vi "Read database.vi"(0 "table":string="CODMn", 1 "显示项":string[](array[string]), 5 "量程下拉列表":enum16{"低量程", "高量程"}(ring), 11 "error in (no error)":errorcluster caption="错误输入（无错误）") -> (4 "表格":string[][](table), 8 "foretime":string, 10 "lasttime":string, 15 "error out":errorcluster caption="错误输出")   [LabVIEW 2016, in "斯坦道CODcr.lvlib"]
uses:
  <vilib>/addons/database/Connection.llb/DB Tools Open Connec (String).vi
  <vilib>/addons/database/_DB Variant To Data/Database Variant To Data.xnode
  <vilib>/addons/database/NI_Database_API.lvlib
  database/SQLite/SQLite Lib.lvlib
  database/Access/Access Lib.lvlib
panel:
  out "电子表格字符串":string
  out "SQL":string="where 时间 between #2020/03/27 14:26:18 # and #2020/04/26 14:26:18# order by 时间 desc"
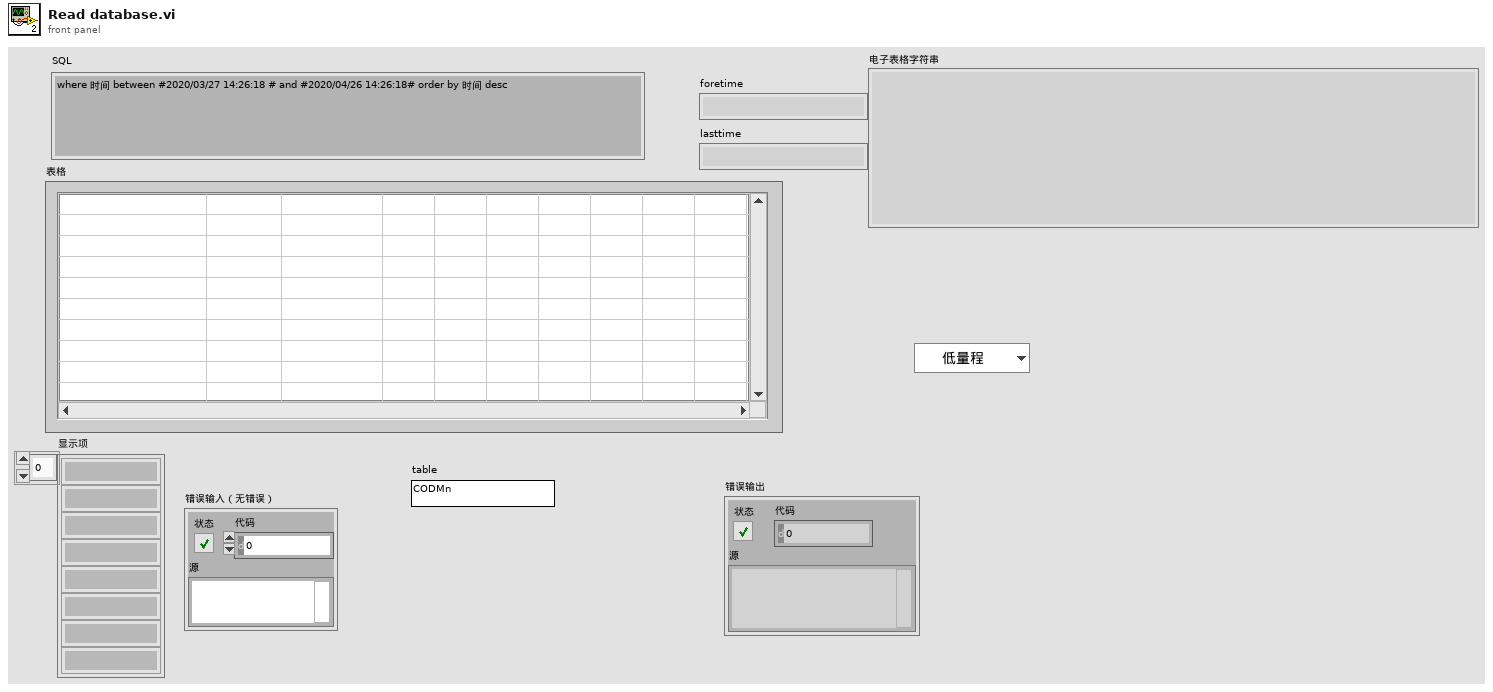
[diagram p1: front panel]
types:
  T1 = typedef "数据库类型.ctl" = enum16{"Access", "SQLite"}
  T2 = typedef "NI_Database_API.lvlib/Conn ObjectReference.ctl" = refnum<k1>
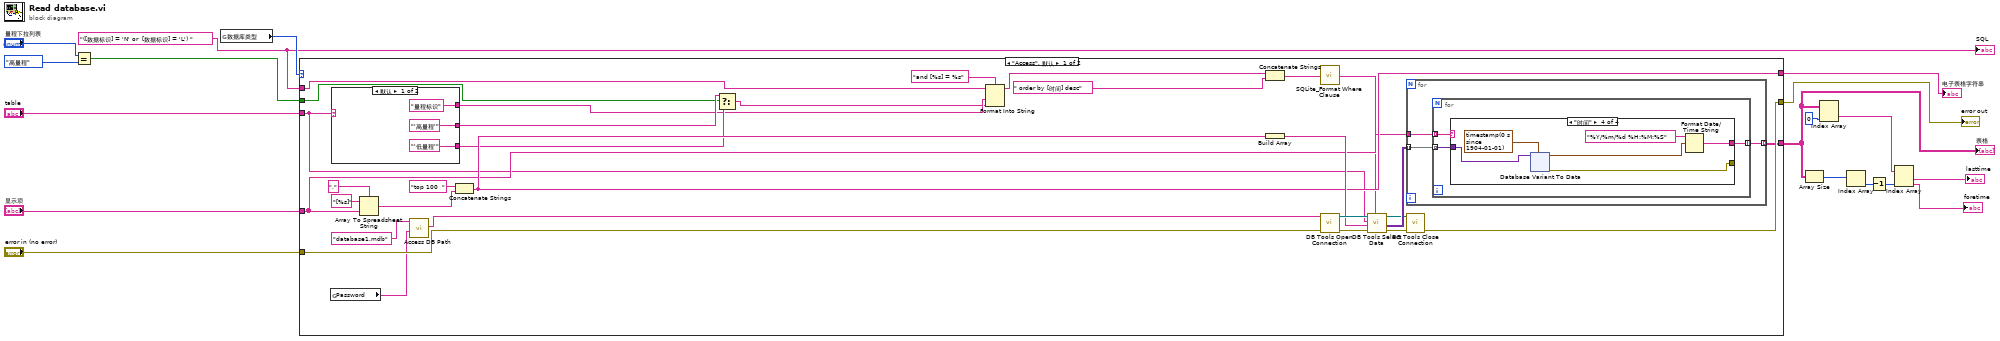
[diagram p0: block diagram]
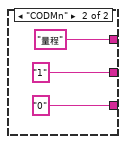
[diagram p2: hidden frame]
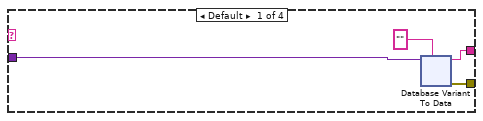
[diagram p3: hidden frame]
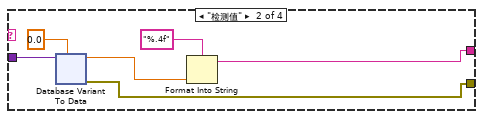
[diagram p4: hidden frame]
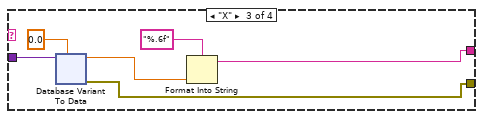
[diagram p5: hidden frame]
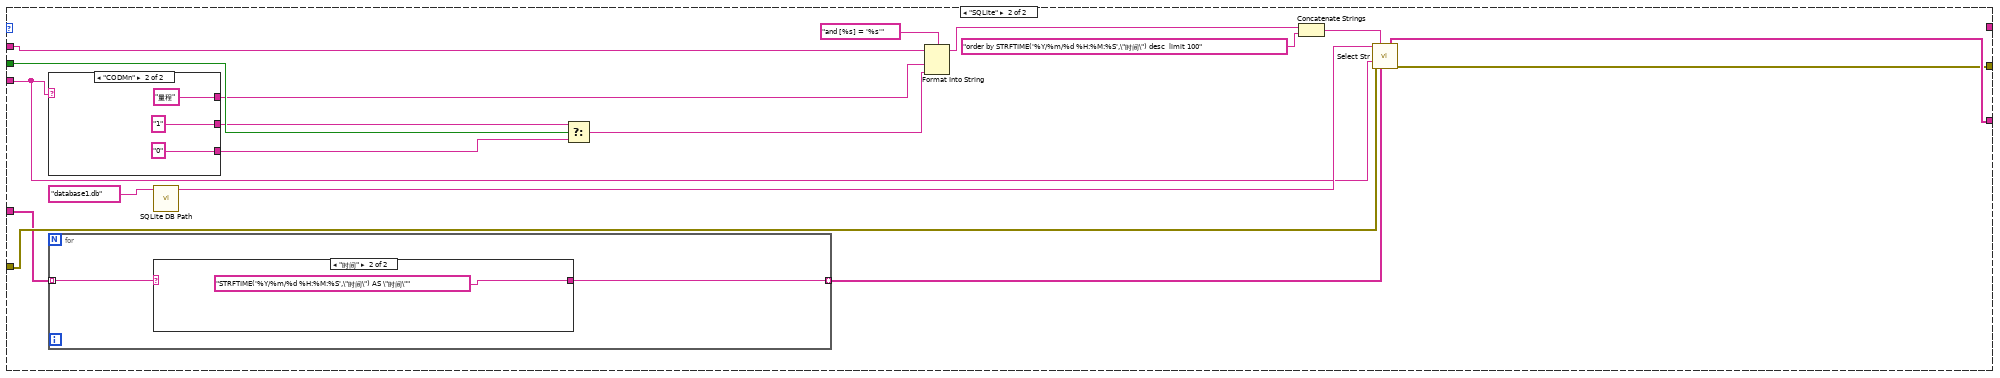
[diagram p6: hidden frame]
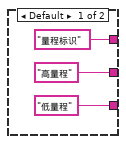
[diagram p7: hidden frame]
diagram:
  w2 = "([数据标识] = 'N' or  [数据标识] = 'L') " ("格式字符串")
  n1 = Equal?(x="量程下拉列表", y=enum16{"低量程", "高量程"}."高量程") -> (x = y?=w1:bool)
  n2 = global read "总磷总氮断电保存全局变量.vi" "数据库类型"() -> (w12:T1)
  n3 = case shown="\"Access\", 默认" w12 {
    tunnel: "error in (no error)" -> [w45 w238]
    tunnel: [w44 w237] -> w17
    tunnel: "table" -> [w24 w232]
    tunnel: [w41 w239] -> w9
    tunnel: w2 -> [w28 w228]
    tunnel: "显示项" -> [w33 w236]
    tunnel: [w34 _] -> w10
    tunnel: w1 -> [w22 w231]
    frame "Access", Default {
      n4 = global read "总磷总氮断电保存全局变量.vi" "Password"() -> (w20:string)
      n5 = case shown="默认" w24 {
        tunnel: ["量程标识" "量程"] -> w23
        tunnel: ["'高量程'" "1"] -> w25
        tunnel: ["'低量程'" "0"] -> w26
        frame Default {
        }
        frame "CODMn" {
        }
      }
      n6 = Array To Spreadsheet String(delimiter (Tab)="," ("分隔符(Tab)"), array=w33, 3:"[%s]" ("格式字符串")) -> (spreadsheet string=w38:string)
      n7 = call "Access DB Path.vi"("Password"=w20, "database"="database1.mdb") -> ("Connection information"=w19:string)  [unwired: 8 in, 1 out]
      n8 = Concatenate Strings("top 100  " ("字符串"), w38) -> (w34:string)
      n9 = Select(t=w25, s=w22, f=w26) -> (s? t:f=w21:string)
      n10 = Format Into String(format string="and [%s] = %s" ("格式字符串"), initial string=w28, w23, w21) -> (resulting string=w29:string)  [unwired: 1 in, 1 out]
      n11 = Concatenate Strings(w29, " order by [时间] desc" ("字符串")) -> (w31:string)
      n12 = Build Array(w34) -> (w35:string[])
      n13 = call <userlib>:"SQLite_Format Where Clause.vi"("Where clause"=w31) -> ("String"=w32:string)  [unwired: 4 in]
      n14 = call-poly <vilib>:"DB Tools Open Connection.vi"("error in (no error)"=w45, "connection information"=w19) -> ("error out"=w47:errorcluster, "connection reference"=w48:T2)  [unwired: 6 in]
      n15 = call <vilib>:"DB Tools Select Data.vi"("condition"=w32, "error in (no error)"=w47, "columns"=w35, "table"=w24, "connection reference"=w48) -> ("error out"=w46:errorcluster, "data"=w43:variant[][], "connection reference out"=w42:T2)  [unwired: 1 in]
      n16 = for {
        tunnel: w43 -> [w57] mode=indexing
        tunnel: [w56] -> w41 mode=indexing
        tunnel: w33 -> [w55]
        n17 = for {
          tunnel: w57 -> [w59] mode=indexing
          tunnel: [w60] -> w56 mode=indexing
          tunnel: w55 -> [w58] mode=indexing
          n18 = case shown="\"时间\"" w58 {
            tunnel: w59 -> [w64 w102 w140 w178]
            tunnel: [w61 w98 w136 w174] -> w60
            tunnel: [w62 w101 w139 w173] -> _
            frame Default {
              n19 = xnode "Database Variant To Data"("database variant"=w64, "type"="") -> ("data"=w61:string, "error out"=w62:errorcluster)  [unwired: 1 in]
            }
            frame "检测值" {
              n20 = xnode "Database Variant To Data"("database variant"=w102, "type"=0.0) -> ("data"=w99:dbl, "error out"=w101:errorcluster)  [unwired: 1 in]
              n21 = Format Into String(format string="%.4f" ("格式字符串"), w99) -> (resulting string=w98:string)  [unwired: 2 in, 1 out]
            }
            frame "X" {
              n22 = xnode "Database Variant To Data"("database variant"=w140, "type"=0.0) -> ("data"=w137:dbl, "error out"=w139:errorcluster)  [unwired: 1 in]
              n23 = Format Into String(format string="%.6f" ("格式字符串"), w137) -> (resulting string=w136:string)  [unwired: 2 in, 1 out]
            }
            frame "时间" {
              n24 = xnode "Database Variant To Data"("database variant"=w178, "type"=timestamp(0 s since 1904-01-01) ("当前时间")) -> ("data"=w177:timestamp, "error out"=w173:errorcluster)  [unwired: 1 in]
              n25 = Format Date/Time String(time format string (%c)="%Y/%m/%d %H:%M:%S" ("时间格式字符串(%c)"), seconds (now)=w177) -> (date/time string=w174:string)  [unwired: 1 in]
            }
          }
        }
      }
      n26 = call <vilib>:"DB Tools Close Connection.vi"("error in (no error)"=w46, "connection reference"=w42) -> ("error out"=w44:errorcluster)  [unwired: 5 in]
    }
    frame "SQLite" {
      n27 = case shown="\"CODMn\"" w232 {
        tunnel: ["量程标识" "量程"] -> w227
        tunnel: ["高量程" "1"] -> w230
        tunnel: ["低量程" "0"] -> w229
        frame Default {
        }
        frame "CODMn" {
        }
      }
      n28 = for {
        tunnel: w236 -> [w249] mode=indexing
        tunnel: [w248] -> w235 mode=indexing
        n29 = case shown="\"时间\"" w249 {
          selector: w249 -> [w250 _]
          tunnel: [w250 "STRFTIME('%Y/%m/%d %H:%M:%S',\"时间\") AS \"时间\""] -> w248
          frame Default {
          }
          frame "时间" {
          }
        }
      }
      n30 = call "SQLite DB Path.vi"("database"="database1.db") -> ("Path out"=w240:string)  [unwired: 10 in]
      n31 = Select(t=w230, s=w231, f=w229) -> (s? t:f=w226:string)
      n32 = Format Into String(format string="and [%s] = '%s'" ("格式字符串"), initial string=w228, w227, w226) -> (resulting string=w224:string)  [unwired: 1 in, 1 out]
      n33 = Concatenate Strings(w224, "order by STRFTIME('%Y/%m/%d %H:%M:%S',\"时间\") desc  limit 100") -> (w234:string)
      n34 = call "Select Str.vi"("DB Path"=w240, "Where Clause"=w234, "Tables Name"=w232, "error in (no error)"=w238, "Columns"=w235) -> ("Results"=w239:string[][], "error out"=w237:errorcluster)  [unwired: 7 in, 2 out]
    }
  }
  "表格" <- w9
  "error out" <- w17
  "电子表格字符串" <- w10
  n35 = Array Size(array=w9) -> (size(s)=w8:i32[])
  n36 = Index Array(array=w9, index (col)=0 ("禁用的索引 (列)")) -> (element=w15:string[])  [unwired: 1 in]
  n37 = Index Array(array=w8) -> (element=w7:i32)  [unwired: 1 in]
  n38 = Decrement(x=w7) -> (x-1=w6:i32)
  n39 = Index Array(array=w15, index #2=w6) -> (element #1=→"lasttime":string, element #2=→"foretime":string)  [unwired: 1 in]
  "SQL" <- w2
